vi "Nufern_controller.vi"() -> ()   [LabVIEW 2014]
uses:
  <vilib>/FieldPoint/Polymorphic Read.llb/FP Read (Float Array).vi
  <vilib>/FieldPoint/Polymorphic Write.llb/FP Write (Float).vi
panel:
  in  "COM Port":string="COM4"
  in  "Controller Stop":bool
  in  "Control Rate (ms)":u32=1000
  in  "AMPLIFIER ENABLE":bool
  in  "LEVEL CONTROL, 0-10 (W)":dbl(knob)=1.0 scale=0.0..10.0
  out "Pre-amp Mon (Amps)":dbl=5.782406330108643 format="%#_3g"
  out "Temp Mon (deg C)":dbl(slide)=24.883191287517548 scale=0.0..50.0
  out "Mid Power Mon (Volts, no-cal)":dbl=4.550704002380371 format="%#_3g"
  out "Out Power Mon (Volts, no-cal)":dbl=1.5106858015060425 format="%#_3g"
  out "+5 Vdc Out":dbl=4.966402530670166 format="%#_3g"
  out "Power-Amp Pump Current (Amps)":dbl format="%#_3g"
  out "Seed Mon (Volts, no-cal)":dbl=4.966084957122803 format="%#_3g"
  out "Back Refl. Mon (Volts, no-cal)":dbl=0.007061874959617853 format="%#_3g"
  out "Power Supply Fault":bool=TRUE
  out "Temp. Fault":bool=TRUE
  out "Back Refl. Fault":bool=TRUE
  out "Seed Power Fault":bool=TRUE
  out "Master Fault":bool=TRUE
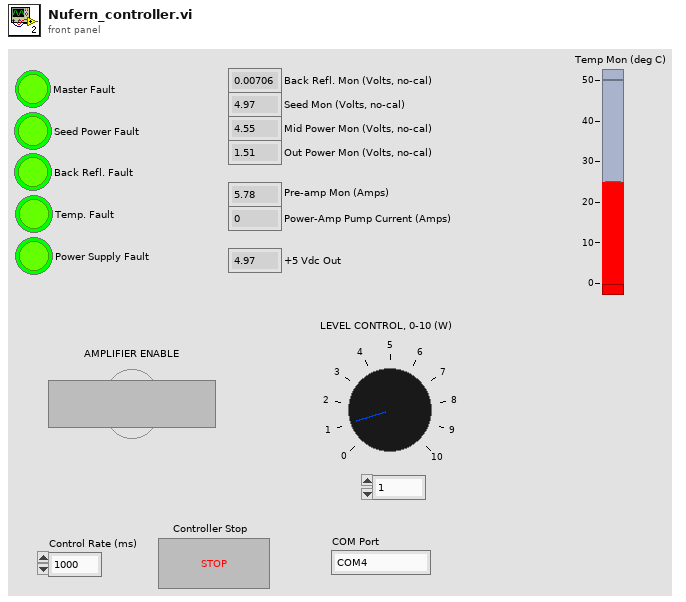
[diagram p1: front panel]
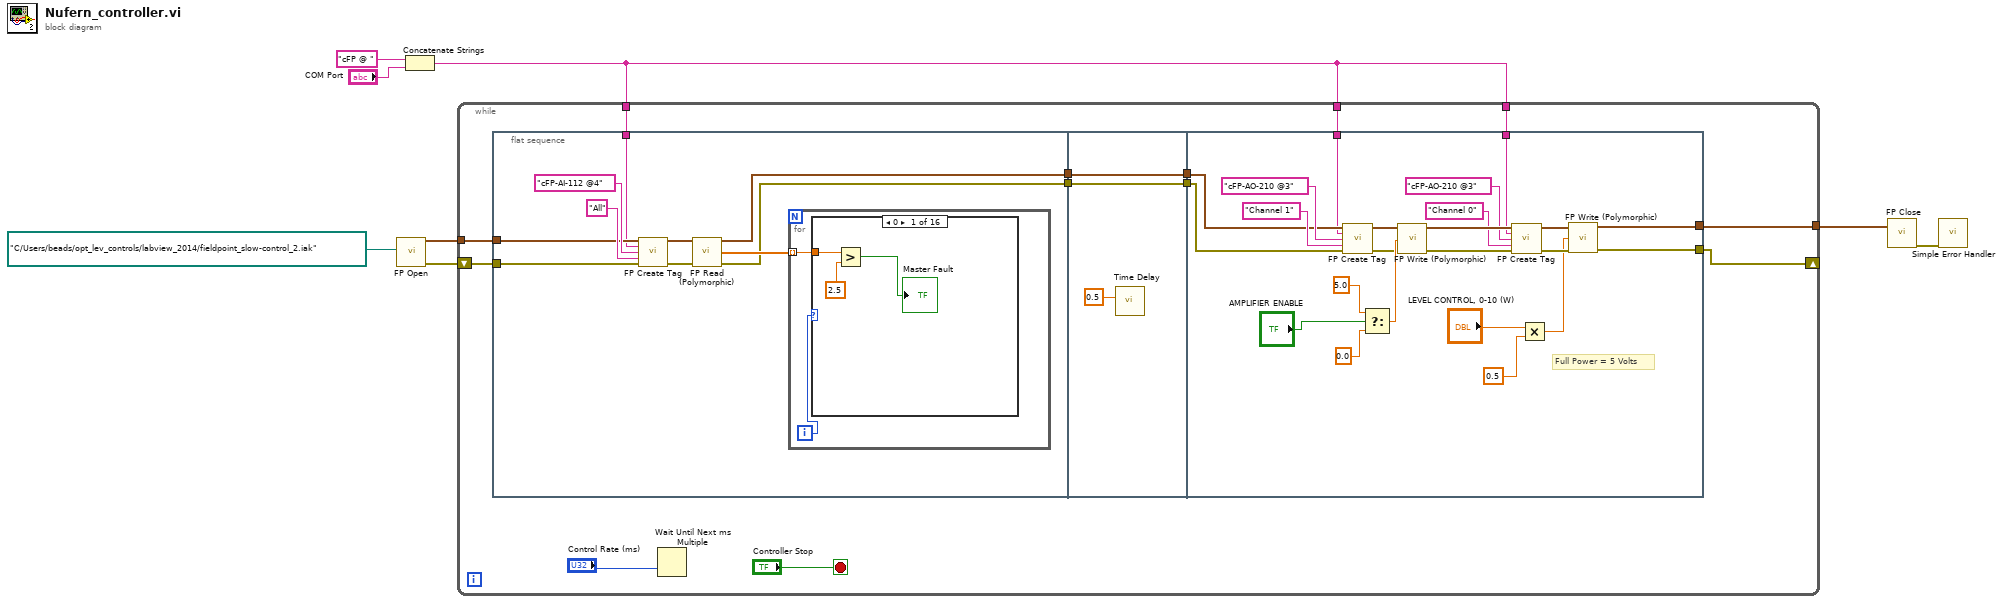
[diagram p0: block diagram]
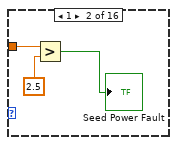
[diagram p2: hidden frame]
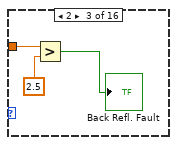
[diagram p3: hidden frame]
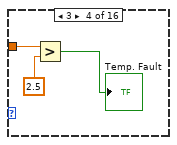
[diagram p4: hidden frame]
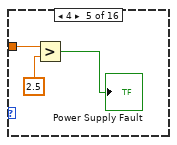
[diagram p5: hidden frame]
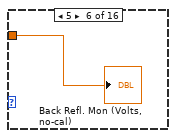
[diagram p6: hidden frame]
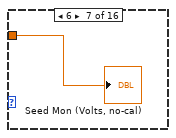
[diagram p7: hidden frame]
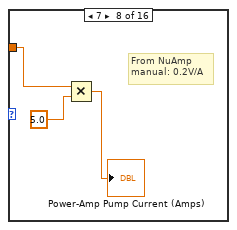
[diagram p8: hidden frame]
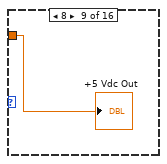
[diagram p9: hidden frame]
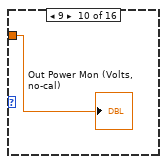
[diagram p10: hidden frame]
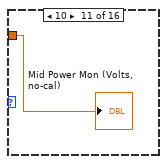
[diagram p11: hidden frame]
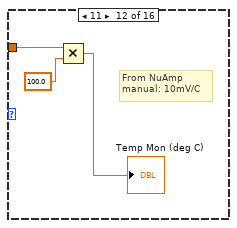
[diagram p12: hidden frame]
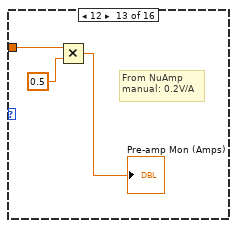
[diagram p13: hidden frame]
diagram:
  n1 = call <vilib>:"FP Open.vi"("iak file path"=path "C:/Users/beads/opt_lev_controls/labview_2014/fieldpoint_slow-control_2.iak") -> ("FP refnum out"=w8:cluster{"server refnum":u32, "tag refnum":u32}, "error out"=w7:errorcluster)  [unwired: 13 in]
  n2 = Concatenate Strings("cFP @ " ("string"), "COM Port") -> (w1:string)
  n3 = while {
    tunnel: w8 -> [w19]
    tunnel: [w17] -> w5
    shift-right: [w16] -> _
    shift-left: w7 -> [w18]
    tunnel: w1 -> [w11]
    tunnel: w1 -> [w10]
    tunnel: w1 -> [w9]
    stop <- "Controller Stop" stop-if-true
    n4 = flat-sequence {
      tunnel: w19 -> [w26]
      tunnel: w18 -> [w25]
      tunnel: [w24] -> w15
      tunnel: [w23] -> w13
      tunnel: w11 -> [w22]
      tunnel: w15 -> [w65]
      tunnel: [w65] -> w14
      tunnel: w13 -> [w64]
      tunnel: [w64] -> w12
      tunnel: w14 -> [w86]
      tunnel: w12 -> [w85]
      tunnel: [w72] -> w17
      tunnel: [w71] -> w16
      tunnel: w10 -> [w67]
      tunnel: w9 -> [w66]
      frame #0 {
        n5 = call <vilib>:"FP Create Tag.vi"("FP refnum in"=w26, "comm resource name"=w22, "device name"="cFP-AI-112 @4" ("Device Name"), "item name"="All" ("Item Name"), "error in (no error)"=w25) -> ("FP refnum out"=w28:cluster{"server refnum":u32, "tag refnum":u32}, "error out"=w27:errorcluster)  [unwired: 9 in]
        n6 = call-poly <vilib>:"FP Read (Polymorphic).vi"("FP refnum in"=w28, "error in (no error)"=w27) -> ("FP refnum out"=w24:cluster{"server refnum":u32, "tag refnum":u32}, "values"=w31:dbl[], "error out"=w23:errorcluster)  [unwired: 10 in, 1 out]
        n7 = for {
          tunnel: w31 -> [w33] mode=indexing
          i -> [w32]
          n8 = case shown="0" w32 {
            tunnel: w33 -> [w36 w39 w42 w45 w48 w49 w50 w53 w54 w55 w56 w58 w61 _ _ _]
            frame 0 {
              n9 = Greater?(x=w36, y=2.5) -> (0:→"Master Fault":bool)
            }
            frame 1 {
              n10 = Greater?(x=w39, y=2.5) -> (0:→"Seed Power Fault":bool)
            }
            frame 2 {
              n11 = Greater?(x=w42, y=2.5) -> (0:→"Back Refl. Fault":bool)
            }
            frame 3 {
              n12 = Greater?(x=w45, y=2.5) -> (0:→"Temp. Fault":bool)
            }
            frame 4 {
              n13 = Greater?(x=w48, y=2.5) -> (0:→"Power Supply Fault":bool)
            }
            frame 5 {
              "Back Refl. Mon (Volts, no-cal)" <- w49
            }
            frame 6 {
              "Seed Mon (Volts, no-cal)" <- w50
            }
            frame 7 {
              # "From NuAmp \nmanual: 0.2V/A"
              n14 = Multiply(x=w53, y=5.0) -> (x*y=→"Power-Amp Pump Current (Amps)":dbl)
            }
            frame 8 {
              "+5 Vdc Out" <- w54
            }
            frame 9 {
              "Out Power Mon (Volts, no-cal)" <- w55
            }
            frame 10 {
              "Mid Power Mon (Volts, no-cal)" <- w56
            }
            frame 11 {
              # "From NuAmp \nmanual: 10mV/C"
              n15 = Multiply(x=w58, y=100.0) -> (x*y=→"Temp Mon (deg C)":dbl)
            }
            frame 12 {
              # "From NuAmp \nmanual: 0.2V/A"
              n16 = Multiply(x=w61, y=0.5) -> (x*y=→"Pre-amp Mon (Amps)":dbl)
            }
            frame 13, Default {
            }
            frame 14 {
            }
            frame 15 {
            }
          }
        }
      }
      frame #1 {
        n17 = call "Time Delay"("Delay Time (s)"=0.5) -> ()  [unwired: 10 in, 1 out]
      }
      frame #2 {
        # "Full Power = 5 Volts"
        n18 = call <vilib>:"FP Create Tag.vi"("FP refnum in"=w86, "comm resource name"=w67, "device name"="cFP-AO-210 @3" ("Device Name"), "item name"="Channel 1" ("Item Name"), "error in (no error)"=w85) -> ("FP refnum out"=w80:cluster{"server refnum":u32, "tag refnum":u32}, "error out"=w79:errorcluster)  [unwired: 9 in]
        n19 = Select(t=5.0, s="AMPLIFIER ENABLE", f=0.0) -> (s? t:f=w81:dbl)
        n20 = call-poly <vilib>:"FP Write (Polymorphic).vi"("FP refnum in"=w80, "value"=w81, "error in (no error)"=w79) -> ("FP refnum out"=w78:cluster{"server refnum":u32, "tag refnum":u32}, "error out"=w77:errorcluster)  [unwired: 10 in, 1 out]
        n21 = call <vilib>:"FP Create Tag.vi"("FP refnum in"=w78, "comm resource name"=w66, "device name"="cFP-AO-210 @3" ("Device Name"), "item name"="Channel 0" ("Item Name"), "error in (no error)"=w77) -> ("FP refnum out"=w74:cluster{"server refnum":u32, "tag refnum":u32}, "error out"=w73:errorcluster)  [unwired: 9 in]
        n22 = Multiply(x="LEVEL CONTROL, 0-10 (W)", y=0.5) -> (x*y=w68:dbl)
        n23 = call-poly <vilib>:"FP Write (Polymorphic).vi"("FP refnum in"=w74, "value"=w68, "error in (no error)"=w73) -> ("FP refnum out"=w72:cluster{"server refnum":u32, "tag refnum":u32}, "error out"=w71:errorcluster)  [unwired: 10 in, 1 out]
      }
    }
    n24 = Wait Until Next ms Multiple(millisecond multiple="Control Rate (ms)") -> ()  [unwired: 1 out]
  }
  n25 = call <vilib>:"FP Close.vi"("FP refnum in"=w5) -> ("error out"=w6:errorcluster)  [unwired: 14 in]
  n26 = call <vilib>:"Simple Error Handler.vi"("error in (no error)"=w6) -> ()  [unwired: 4 in, 5 out]
